vi "Modbus error wrapper.vi"(2 "Response from correct drive":bool, 3 "Comms error":errorcluster, 4 "Modbus exception code":T1=1 items=["None"=0, "Invalid function request"=1, "Invalid Modbus register address"=2, "Invalid / unauthorised data value"=3, "Device failure"=4, "Request accepted, wait"=5, "Drive busy"=6, "Request rejected"=7, "Memory parity error"=8, "Gateway path unavailable"=10, "Device failed to respond"=11], 5 "Checksum ok":bool) -> (0 "Modbus error cluster":T2={"Checksum ok"=FALSE, "Modbus exception code"=1, "Response from correct drive"=FALSE, "Comms error"={"status"=FALSE, "code"=0, "source"=""}} {"Modbus exception code" items=["None"=0, "Invalid function request"=1, "Invalid Modbus register address"=2, "Invalid / unauthorised data value"=3, "Device failure"=4, "Request accepted, wait"=5, "Drive busy"=6, "Request rejected"=7, "Memory parity error"=8, "Gateway path unavailable"=10, "Device failed to respond"=11]}, 1 "No errors":bool)   [LabVIEW 2020]
doc: "Modbus RTU for Invertek drives. Paul Nathan 21-JUN-2022."
uses:
  ctls/Modbus error cluster.ctl
  ctls/Exception codes.ctl
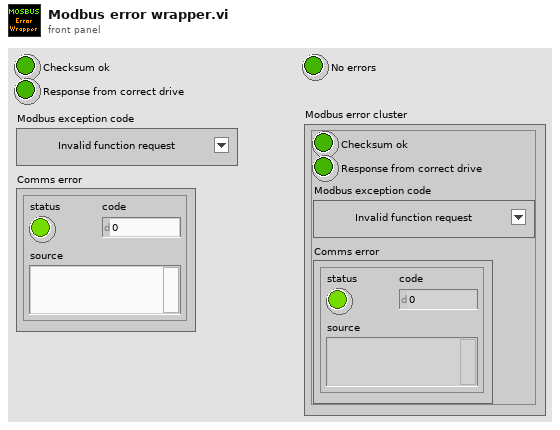
[diagram p1: front panel]
types:
  T1 = typedef "Exception codes.ctl" = u8
  T2 = typedef "Modbus error cluster.ctl" = cluster{"Checksum ok":bool, "Modbus exception code":T1, "Response from correct drive":bool, "Comms error":errorcluster}
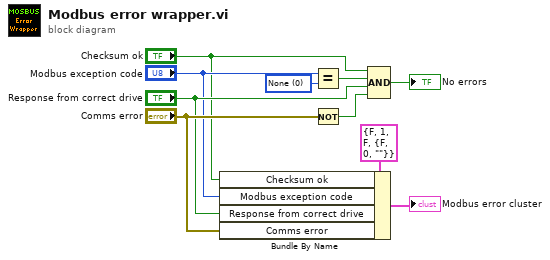
[diagram p0: block diagram]
diagram:
  w10 = T1 0 items=["None"=0, "Invalid function request"=1, "Invalid Modbus register address"=2, "Invalid / unauthorised data value"=3, "Device failure"=4, "Request accepted, wait"=5, "Drive busy"=6, "Request rejected"=7, "Memory parity error"=8, "Gateway path unavailable"=10, "Device failed to respond"=11] ("y")
  n1 = Bundle By Name(cluster=T2 {"Checksum ok"=FALSE, "Modbus exception code"=1, "Response from correct drive"=FALSE, "Comms error"={"status"=FALSE, "code"=0, "source"=""}} ("Modbus error cluster"), "Checksum ok"="Checksum ok", "Modbus exception code"="Modbus exception code", "Response from correct drive"="Response from correct drive", "Comms error"="Comms error") -> (→"Modbus error cluster":T2)
  n2 = Equal?(x="Modbus exception code", y=w10) -> (x = y?=w9:bool)
  n3 = Not(x="Comms error") -> (.not. x?=w8:bool)
  n4 = Compound Arithmetic op=AND("Checksum ok", w9, "Response from correct drive", w8) -> (→"No errors":bool)
